vi "Close Plugin SubPanels from Map.vi"(8 "error in (no error)":errorcluster, 11 "CIF_UI in":refnum<class "CIF_UI.lvclass">) -> (0 "error out":errorcluster, 3 "CIF_UI out":refnum<class "CIF_UI.lvclass">)   [LabVIEW 2021, in "CIF_UI.lvclass"]
uses:
  CIF_UI.lvclass
  Typedef/Plugin Subpanel Map.ctl
  Typedef/Subpanel Data.ctl
  Typedef/Plugin Subpanel Events.ctl
  CIF_UI.lvclass/CIF_UI.ctl
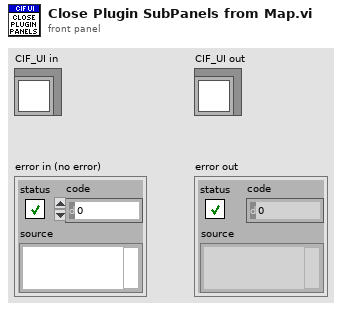
[diagram p1: front panel]
types:
  T1 = typedef "CIF_UI.lvclass/Plugin Subpanel Map.ctl" = map{i32, T2}
  T2 = typedef "CIF_UI.lvclass/Subpanel Data.ctl" = cluster{"VI Reference":refnum<vi>, "Plugin Subpanel Events":T3}
  T3 = typedef "CIF_UI.lvclass/Plugin Subpanel Events.ctl" = cluster{"Plugin Shutdown":refnum<user-event>}
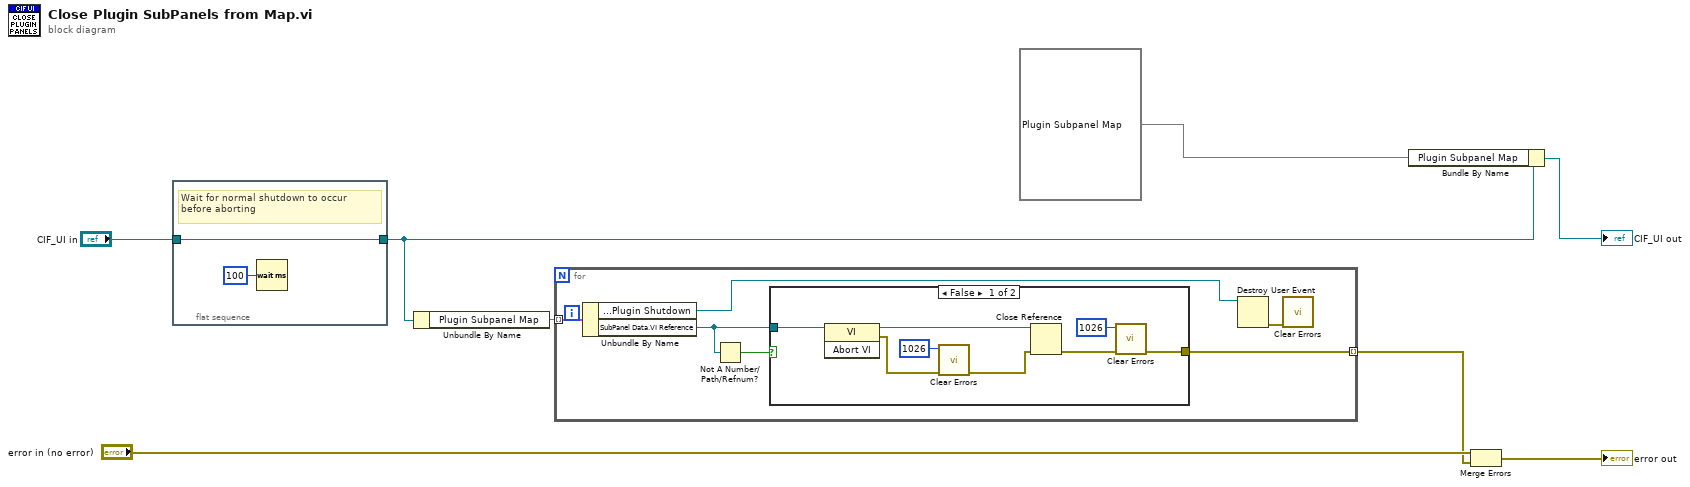
[diagram p0: block diagram]
diagram:
  n1 = flat-sequence {
    tunnel: "CIF_UI in" -> [w9]
    tunnel: [w9] -> w2
    frame #0 {
      # "Wait for normal shutdown to occur before aborting"
      n2 = Wait (ms)(milliseconds to wait=u32 100) -> ()  [unwired: 1 out]
    }
  }
  n3 = Unbundle By Name(w2) -> ("Plugin Subpanel Map"=w7:T1)
  n4 = for {
    tunnel: w7 -> [w16] mode=indexing
    tunnel: [w13] -> w5 mode=indexing
    n5 = Unbundle By Name(w16) -> ("SubPanel Data.Plugin Subpanel Events.Plugin Shutdown"=w12:refnum<user-event>, "SubPanel Data.VI Reference"=w14:refnum<vi>)
    n6 = Not A Number/Path/Refnum?(number/path/refnum=w14) -> (NaN/Path/Refnum?=w15:bool)
    n7 = case shown="False" w15 {
      tunnel: w14 -> [w24 _]
      tunnel: [w17 _] -> w13
      frame False {
        n8 = invoke class="VI" method="Abort VI"(reference=w24) -> (reference out=w23:refnum<vi>, error out=w21:errorcluster)  [unwired: 2 in, 1 out]
        n9 = call <vilib>:"Clear Errors.vi"("error in (no error)"=w21, "specific error code to clear (0: all)"=1026) -> ("error out"=w20:errorcluster)  [unwired: 4 in, 1 out]
        n10 = Close Reference(reference=w23, error in (no error)=w20) -> (error out=w18:errorcluster)
        n11 = call <vilib>:"Clear Errors.vi"("error in (no error)"=w18, "specific error code to clear (0: all)"=1026) -> ("error out"=w17:errorcluster)  [unwired: 4 in, 1 out]
      }
      frame True {
      }
    }
    n12 = Destroy User Event(user event=w12) -> (error out=w11:errorcluster)  [unwired: 1 in]
    n13 = call <vilib>:"Clear Errors.vi"("error in (no error)"=w11) -> ()  [unwired: 5 in, 2 out]
  }
  n14 = Bundle By Name(cluster=w2, "Plugin Subpanel Map"=T1 {}) -> (→"CIF_UI out":refnum<class "CIF_UI.lvclass">)
  n15 = Merge Errors("error in (no error)", w5) -> (→"error out":errorcluster)
